vi "Load-sequences.vi"(8 "error in (no error)":errorcluster, 11 "Available motors in":refnum<class "Motor-assembly.lvclass">) -> (0 "error out":errorcluster, 3 "Available motors out":refnum<class "Motor-assembly.lvclass">)   [LabVIEW 2013, in "PowderDeposition.lvlib" / "Motor-assembly.lvclass"]
uses:
  Motor-assembly.lvclass
  Motor-assembly.lvclass/Motor-assembly.ctl
  Motor/Motor.lvclass
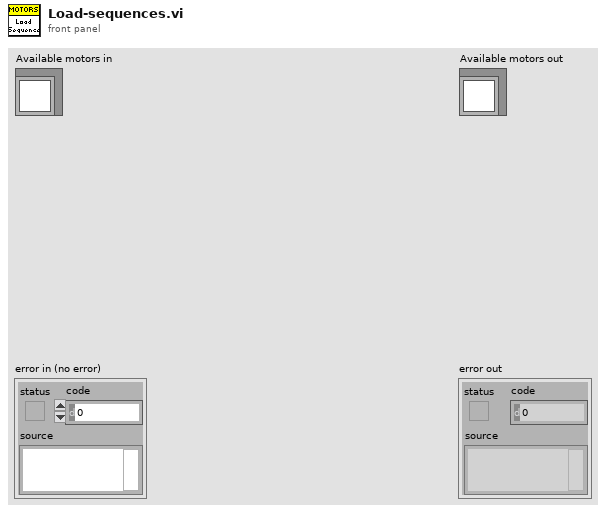
[diagram p1: front panel]
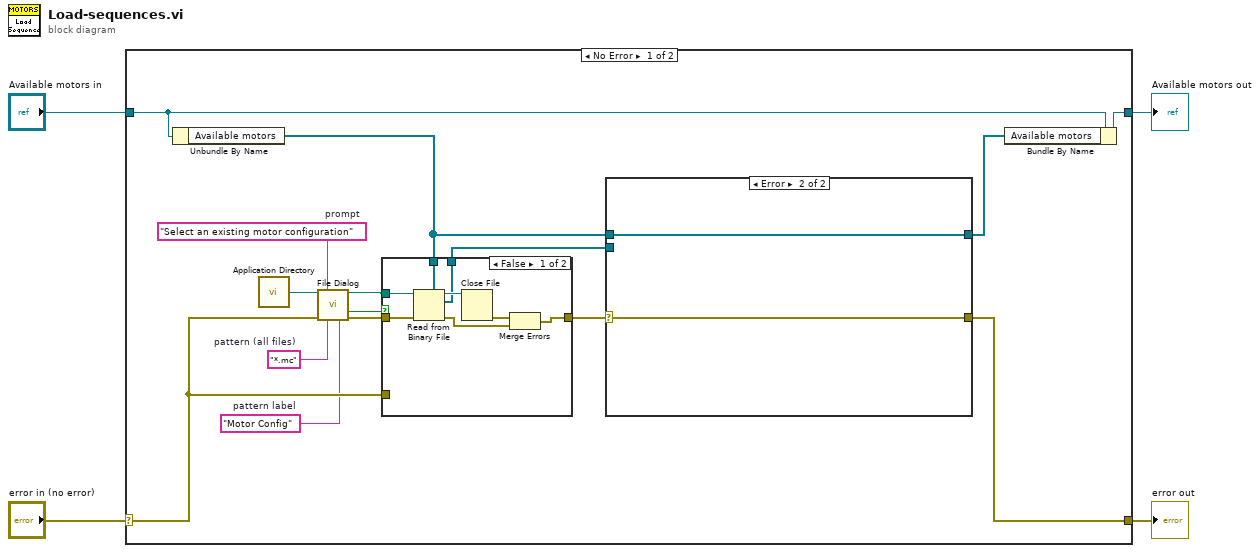
[diagram p0: block diagram]
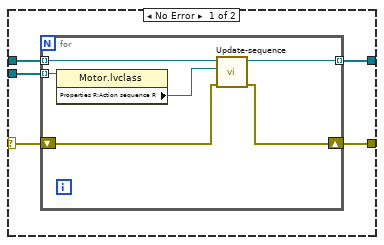
[diagram p2: hidden frame]
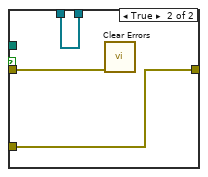
[diagram p3: hidden frame]
diagram:
  n1 = case shown="No Error" "error in (no error)" {
    selector: "error in (no error)" -> [w8 w45]
    tunnel: [w13 w45] -> w3
    tunnel: [w17 w44] -> w1
    tunnel: "Available motors in" -> [w19 w44]
    frame No Error {
      w6 = "Motor Config"  # pattern label
      w7 = "*.mc"  # pattern (all files)
      w10 = "Select an existing motor configuration"  # prompt
      n2 = Unbundle By Name(w19) -> ("Available motors"=w16:refnum<class "Motor.lvclass">[])
      n3 = call <vilib>:"Application Directory.vi"() -> ("Application Directory"=w9:path)
      n4 = call "File Dialog"("start path"=w9, "prompt"=w10, "error in"=w8, "pattern (all files)"=w7, "pattern label"=w6) -> ("selected path"=w18:path, "cancelled"=w11:bool, "error out"=w12:errorcluster)  [unwired: 7 in, 1 out]
      n5 = case shown="False" w11 {
        tunnel: w12 -> [w40 w41]
        tunnel: w18 -> [w39 _]
        tunnel: w16 -> [w38 w43]
        tunnel: [w36 w43] -> w15
        tunnel: [w35 w42] -> w5
        tunnel: w8 -> [_ w42]
        frame False {
          n6 = Read from Binary File(5:w38, 8:w40, 11:w39) -> (0:w33:errorcluster, 2:w36:refnum<class "Motor.lvclass">[], 3:w37:refnum<file>)  [unwired: 3 in, 1 out]
          n7 = Close File(refnum=w37) -> (error out=w34:errorcluster)  [unwired: 1 in, 1 out]
          n8 = Merge Errors(w34, w33) -> (w35:errorcluster)
        }
        frame True {
          n9 = call <vilib>:"Clear Errors.vi"("error in (no error)"=w41) -> ()  [unwired: 6 in, 1 out]
        }
      }
      n10 = case shown="Error" w5 {
        selector: w5 -> [w20 w31]
        tunnel: w16 -> [w24 w32]
        tunnel: w15 -> [w23 _]
        tunnel: [w22 w32] -> w14
        tunnel: [w21 w31] -> w13
        frame No Error {
          n11 = for {
            tunnel: w23 -> [w30] mode=indexing
            tunnel: w24 -> [w29] mode=indexing
            tunnel: [w27] -> w22 mode=indexing
            shift-right: [w25] -> w21
            shift-left: w20 -> [w26]
            n12 = property class="Motor.lvclass"(reference=w30) -> ("Properties R:Action sequence R"=w28:refnum<class "Action-sequence.lvclass">)  [unwired: 1 in, 2 out]
            n13 = call-dynamic "Update-sequence.vi"("error in (no error)"=w26, "Sequence"=w28, "Motor in"=w29) -> ("error out"=w25:errorcluster, "Motor out"=w27:refnum<class "Motor.lvclass">)  [unwired: 7 in]
          }
        }
        frame Error {
        }
      }
      n14 = Bundle By Name(cluster=w19, "Available motors"=w14) -> (w17:refnum<class "Motor-assembly.lvclass">)
    }
    frame Error {
    }
  }
  "error out" <- w3
  "Available motors out" <- w1
